vi "Get Inset Image JPG Name.vi"(4 "Inset Data Path":path, 5 "Inkscape Path":path) -> (1 "Inset JPG Name":string)   [LabVIEW 2019]
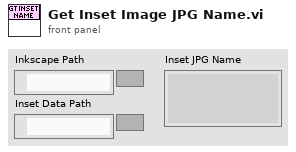
[diagram p1: front panel]
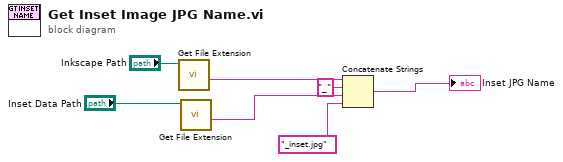
[diagram p0: block diagram]
diagram:
  n1 = call <vilib>:"Get File Extension.vi"("file"="Inkscape Path") -> ("filename without extension"=w7:string)  [unwired: 6 in, 4 out]
  n2 = call <vilib>:"Get File Extension.vi"("file"="Inset Data Path") -> ("filename without extension"=w1:string)  [unwired: 6 in, 4 out]
  n3 = Concatenate Strings(w7, "_" ("string"), w1, "_inset.jpg" ("string")) -> (→"Inset JPG Name":string)
